vi "Read DC meter.vi"(6 "No of readings":i32=1, 7 "abort reference":refnum<vi>, 8 "error in (no error)":errorcluster, 11 "DC meter":T1={"DC meter type"=enum."H/A/K 3458", "DC meter VISA"="", "NPLC"=10.0, "status ref"=refnum}) -> (0 "error out":errorcluster, 2 "DC readings":dbl[](array[numeric]), 3 "DC meter out":T1={"DC meter type"=enum."H/A/K 3458", "DC meter VISA"="", "NPLC"=10.0, "status ref"=refnum})   [LabVIEW 2020]
doc: "Read selected number of values from the DC meter."
uses:
  Type definitions/DC meter.ctl
  Type definitions/DC meter type.ctl
  <vilib>/Utility/error.llb/Error Cluster From Error Code.vi
  external libraries/3458A Basic Driver/Public/Data/Read Measurement(Single Point).vi
  <vilib>/ErrorRing/Error Ring.xnode
  external libraries/Fluke 8508/Fluke 8508.lvlib
  external libraries/3458A Basic Driver/3458A Basic Driver.lvlib
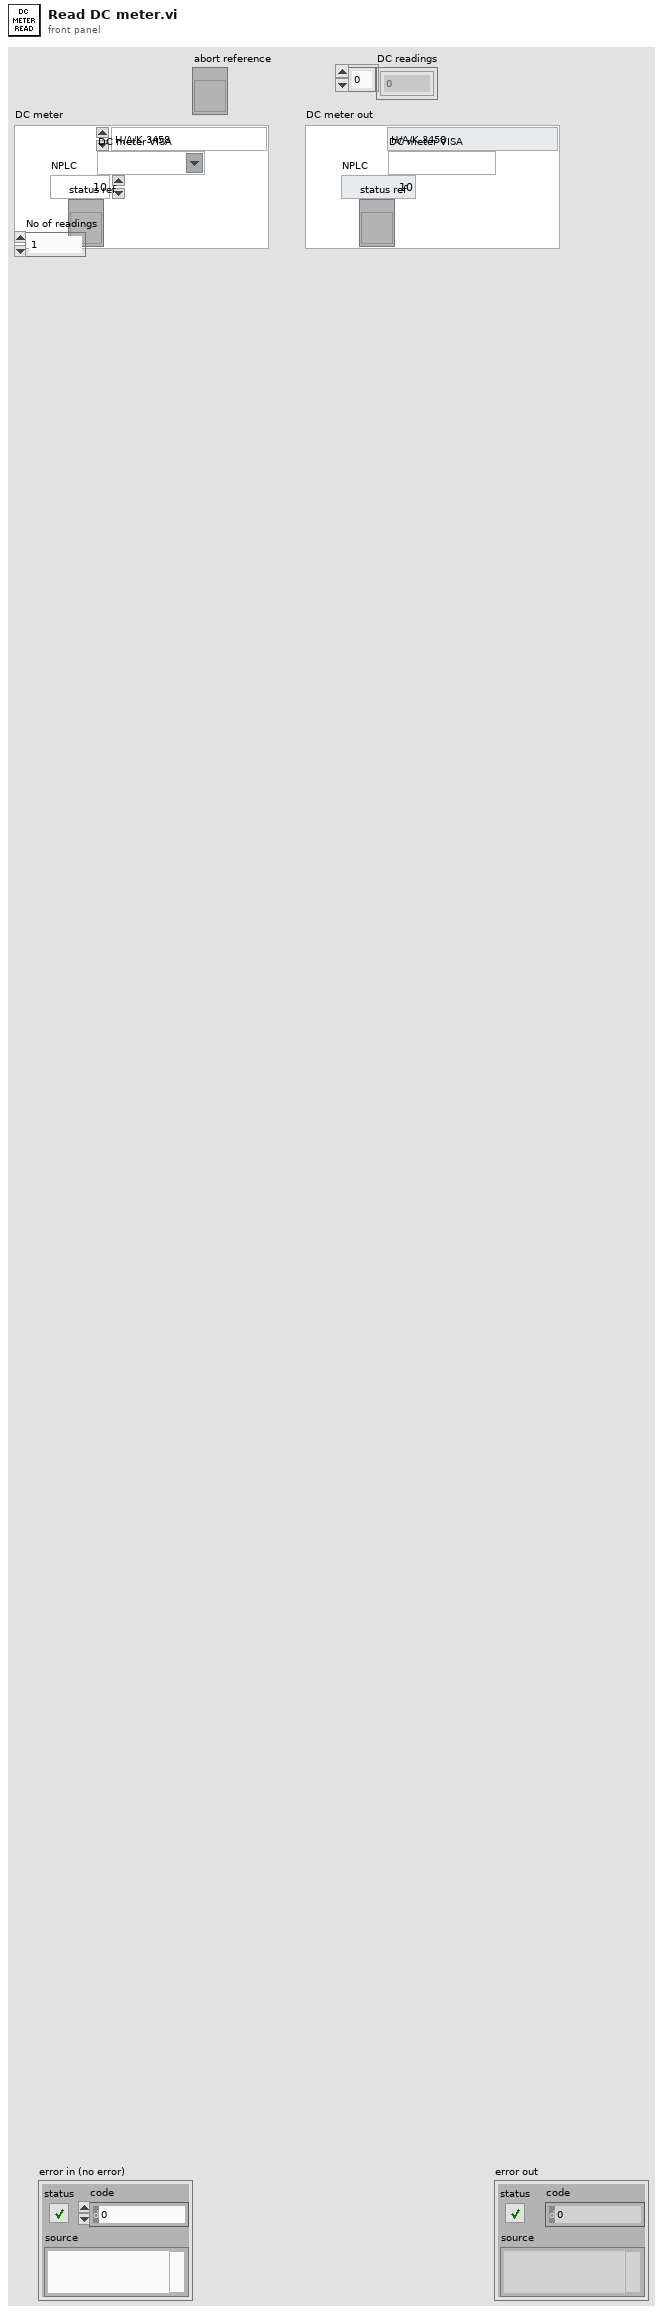
[diagram p1: front panel]
types:
  T1 = typedef "DC meter.ctl" = cluster{"DC meter type":T2, "DC meter VISA":refnum<visa-resource-name>, "NPLC":dbl, "status ref":refnum<vi>}
  T2 = typedef "DC meter type.ctl" = enum16{"H/A/K 3458", "Fluke 8508A", "dummy", "Keithley 2182"}
  T3 = cluster{"error":bool, "code":i32, "source":string}
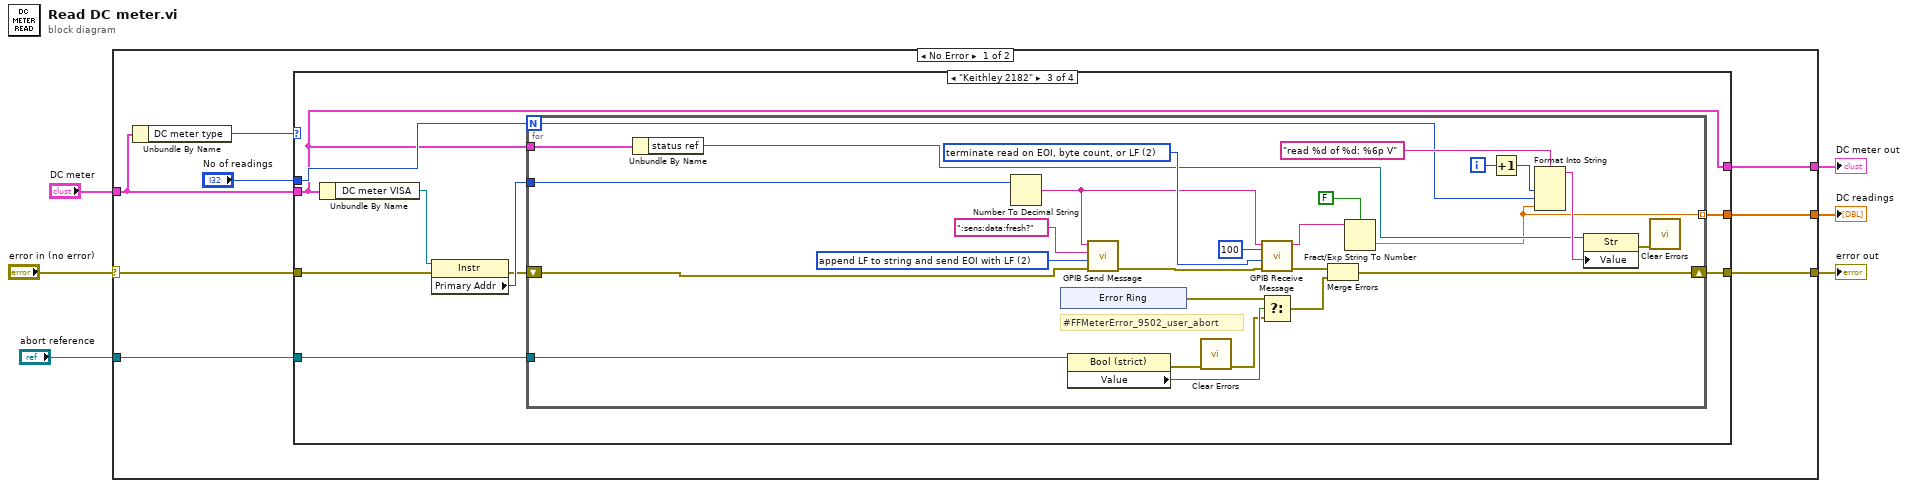
[diagram p0: block diagram]
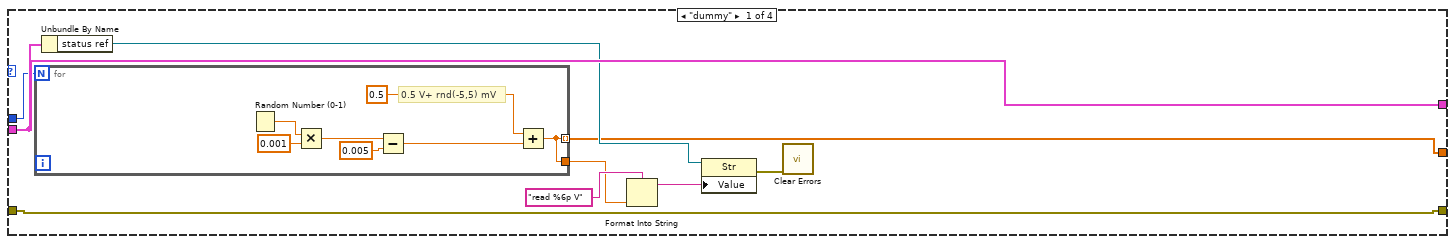
[diagram p2: hidden frame]
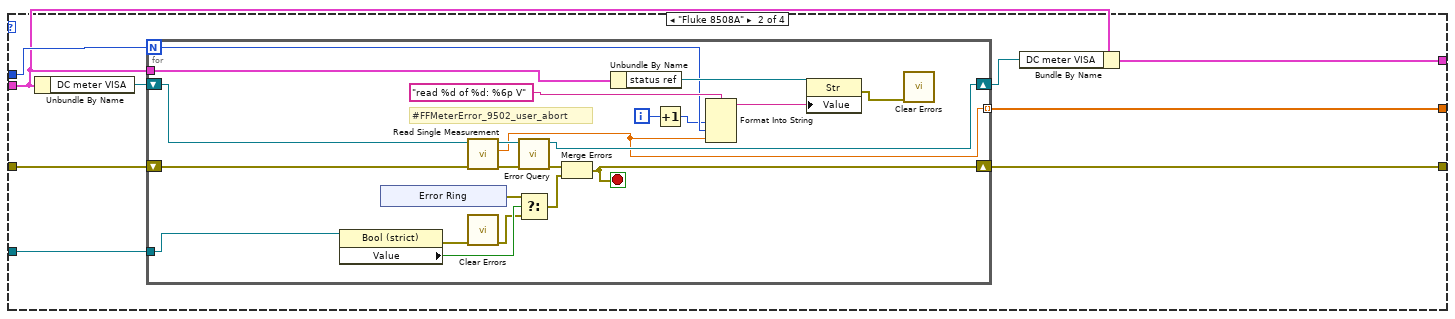
[diagram p3: hidden frame]
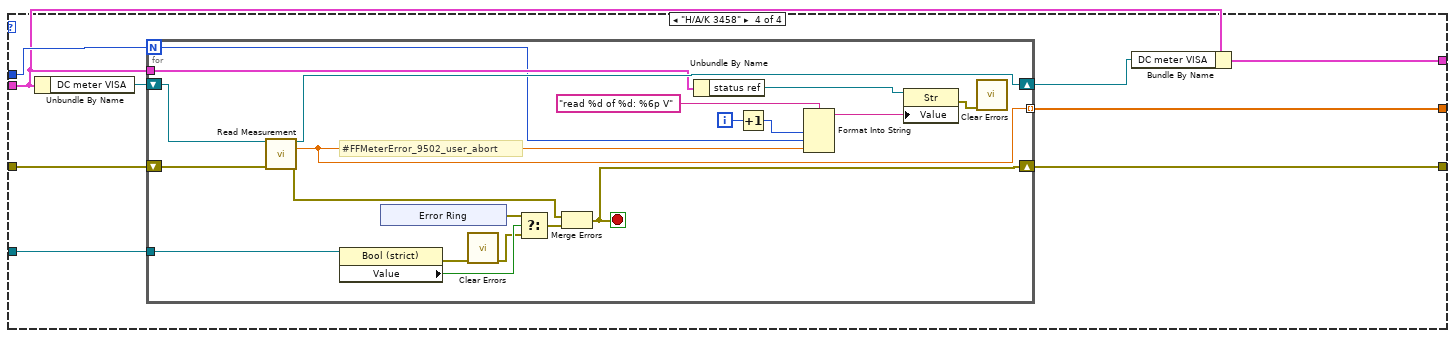
[diagram p4: hidden frame]
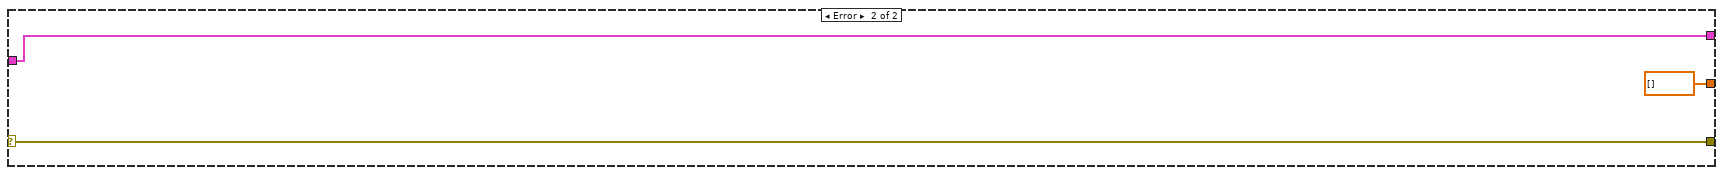
[diagram p5: hidden frame]
diagram:
  n1 = case shown="No Error" "error in (no error)" {
    selector: "error in (no error)" -> [w10 w144]
    tunnel: [w14 w144] -> w6
    tunnel: "DC meter" -> [w12 w143]
    tunnel: [w9 w143] -> w4
    tunnel: [w11 dbl[] [] ("Measurements")] -> w3
    tunnel: "abort reference" -> [w8 _]
    frame No Error {
      n2 = Unbundle By Name(w12) -> ("DC meter type"=w13:T2)
      n3 = case shown="\"Keithley 2182\"" w13 {
        tunnel: w10 -> [w23 w39 w74 w116]
        tunnel: [w23 w36 w71 w115] -> w14
        tunnel: w12 -> [w19 w33 w68 w110]
        tunnel: [w19 w37 w68 w109] -> w9
        tunnel: [w16 w32 w67 w113] -> w11
        tunnel: "No of readings" -> [w17 w34 w70 w112]
        tunnel: w8 -> [_ w31 w69 w108]
        frame "dummy" {
          n4 = for {
            N: w17 -> [_]
            tunnel: [w24] -> w16 mode=indexing
            tunnel: [w24] -> w15
            # "0.5 V+ rnd(-5,5) mV"
            n5 = Random Number (0-1)() -> (number: 0 to 1=w30:dbl)
            n6 = Multiply(x=w30, y=0.001) -> (x*y=w28:dbl)
            n7 = Subtract(x=w28, y=0.005) -> (x-y=w26:dbl)
            n8 = Add(x=0.5, y=w26) -> (x+y=w24:dbl)
          }
          n9 = Unbundle By Name(w19) -> ("status ref"=w18:refnum<vi>)
          n10 = Format Into String(format string="read %6p V", w15) -> (resulting string=w22:string)  [unwired: 2 in, 1 out]
          n11 = property class="Str"(reference=w18, "Value"=w22) -> (error out=w20:errorcluster)  [unwired: 1 in, 1 out]
          n12 = call <vilib>:"Clear Errors.vi"("error in (no error)"=w20) -> ()  [unwired: 5 in, 2 out]
        }
        frame "Fluke 8508A" {
          n13 = Unbundle By Name(w33) -> ("DC meter VISA"=w38:refnum<visa-resource-name>)
          n14 = for {
            N: w34 -> [w43]
            tunnel: [w44] -> w32 mode=indexing
            shift-right: [w40] -> w36
            shift-left: w39 -> [w61]
            shift-right: [w57] -> w35
            shift-left: w38 -> [w60]
            tunnel: w33 -> [w53]
            tunnel: w31 -> [w46]
            i -> [w42]
            stop <- w40 stop-if-true
            # "#FFMeterError_9502_user_abort"
            n15 = property class="Bool (strict)"(reference=w46) -> (error out=w51:errorcluster, "Value"=w50:bool)  [unwired: 1 in, 1 out]
            n16 = xnode "Error Ring"() -> ("error out"=w49:errorcluster)
            n17 = call "Read Single Measurement.vi"("error in (no error)"=w61, "VISA resource name"=w60) -> ("error out"=w59:errorcluster, "Measurement"=w44:dbl, "VISA resource name out"=w58:refnum<visa-resource-name>)  [unwired: 7 in]
            n18 = call <vilib>:"Clear Errors.vi"("error in (no error)"=w51) -> ("error out"=w48:errorcluster)  [unwired: 5 in, 1 out]
            n19 = call "Error Query.vi"("error in (no error)"=w59, "VISA resource name"=w58) -> ("error out"=w45:errorcluster, "VISA resource name out"=w57:refnum<visa-resource-name>)  [unwired: 6 in, 2 out]
            n20 = Select(t=w49, s=w50, f=w48) -> (s? t:f=w47:errorcluster)
            n21 = Merge Errors(w45, w47) -> (w40:errorcluster)
            n22 = Unbundle By Name(w53) -> ("status ref"=w56:refnum<vi>)
            n23 = Increment(x=w42) -> (x+1=w41:i32)
            n24 = Format Into String(format string="read %d of %d: %6p V", w41, w43, w44) -> (resulting string=w52:string)  [unwired: 2 in, 1 out]
            n25 = property class="Str"(reference=w56, "Value"=w52) -> (error out=w55:errorcluster)  [unwired: 1 in, 1 out]
            n26 = call <vilib>:"Clear Errors.vi"("error in (no error)"=w55) -> ()  [unwired: 5 in, 2 out]
          }
          n27 = Bundle By Name(cluster=w33, "DC meter VISA"=w35) -> (w37:T1)
        }
        frame "Keithley 2182" {
          n28 = Unbundle By Name(w68) -> ("DC meter VISA"=w75:refnum<visa-resource-name>)
          n29 = property class="Instr"(reference=w75, error in=w74) -> (error out=w72:errorcluster, "Primary Addr"=w73:u16)  [unwired: 1 out]
          n30 = for {
            N: w70 -> [w78]
            tunnel: w73 -> [w102]
            shift-right: [w86] -> w71
            shift-left: w72 -> [w101]
            tunnel: w69 -> [w85]
            tunnel: w68 -> [w77]
            tunnel: [w76] -> w67 mode=indexing
            i -> [w79]
            w96 = 2 items=["terminate read on EOI or byte count", "terminate read on EOI, byte count, or CR", "terminate read on EOI, byte count, or LF"] ("read mode")
            w98 = 2 items=["send EOI with last character of string", "append CR to string and send EOI with CR", "append LF to string and send EOI with LF", "append CR LF to string and send EOI with LF", "append CR to string but do not send EOI", "append LF to string but do not send EOI", "append CR LF to string but do not send EOI", "do not send EOI"] ("write mode (set END:0)")
            # "#FFMeterError_9502_user_abort"
            n31 = Unbundle By Name(w77) -> ("status ref"=w83:refnum<vi>)
            n32 = Number To Decimal String(number=w102) -> (decimal integer string=w94:string)  [unwired: 1 in]
            n33 = xnode "Error Ring"() -> ("error out"=w89:errorcluster)
            n34 = property class="Bool (strict)"(reference=w85) -> (error out=w91:errorcluster, "Value"=w90:bool)  [unwired: 1 in, 1 out]
            n35 = call "GPIB Send Message.vi"("address string"=w94, "write buffer"=":sens:data:fresh?", "write mode (set END:0)"=w98, "error in"=w101) -> ("error out"=w100:T3)  [unwired: 3 in, 2 out]
            n36 = call <vilib>:"Clear Errors.vi"("error in (no error)"=w91) -> ("error out"=w88:errorcluster)  [unwired: 5 in, 1 out]
            n37 = call "GPIB Receive Message.vi"("address string"=w94, "byte count"=100, "read mode"=w96, "error in"=w100) -> ("read buffer"=w93:string, "error out"=w87:T3)  [unwired: 3 in, 1 out]
            n38 = Select(t=w89, s=w90, f=w88) -> (s? t:f=w92:errorcluster)
            n39 = Merge Errors(w87, w92) -> (w86:errorcluster)
            n40 = Fract/Exp String To Number(use system decimal point (T)=FALSE, string=w93) -> (number=w76:dbl)  [unwired: 2 in, 1 out]
            n41 = Increment(x=w79) -> (x+1=w81:i32)
            n42 = Format Into String(format string="read %d of %d: %6p V", w81, w78, w76) -> (resulting string=w84:string)  [unwired: 2 in, 1 out]
            n43 = property class="Str"(reference=w83, "Value"=w84) -> (error out=w82:errorcluster)  [unwired: 1 in, 1 out]
            n44 = call <vilib>:"Clear Errors.vi"("error in (no error)"=w82) -> ()  [unwired: 5 in, 2 out]
          }
        }
        frame "H/A/K 3458" {
          n45 = Unbundle By Name(w110) -> ("DC meter VISA"=w114:refnum<visa-resource-name>)
          n46 = for {
            N: w112 -> [w119]
            tunnel: [w120] -> w113 mode=indexing
            shift-right: [w121] -> w115
            shift-left: w116 -> [w136]
            shift-right: [w130] -> w111
            shift-left: w114 -> [w135]
            tunnel: w110 -> [w129]
            tunnel: w108 -> [w124]
            i -> [w118]
            stop <- w121 stop-if-true
            # "#FFMeterError_9502_user_abort"
            n47 = call-poly "Read Measurement.vi"("VISA resource name"=w135, "error in (no error)"=w136) -> ("VISA resource name out"=w130:refnum<visa-resource-name>, "Measurement"=w120:dbl, "error out"=w123:errorcluster)  [unwired: 11 in]
            n48 = property class="Bool (strict)"(reference=w124) -> (error out=w128:errorcluster, "Value"=w127:bool)  [unwired: 1 in, 1 out]
            n49 = xnode "Error Ring"() -> ("error out"=w126:errorcluster)
            n50 = call <vilib>:"Clear Errors.vi"("error in (no error)"=w128) -> ("error out"=w125:errorcluster)  [unwired: 5 in, 1 out]
            n51 = Select(t=w126, s=w127, f=w125) -> (s? t:f=w122:errorcluster)
            n52 = Merge Errors(w123, w122) -> (w121:errorcluster)
            n53 = Unbundle By Name(w129) -> ("status ref"=w133:refnum<vi>)
            n54 = Increment(x=w118) -> (x+1=w117:i32)
            n55 = Format Into String(format string="read %d of %d: %6p V", w117, w119, w120) -> (resulting string=w134:string)  [unwired: 2 in, 1 out]
            n56 = property class="Str"(reference=w133, "Value"=w134) -> (error out=w132:errorcluster)  [unwired: 1 in, 1 out]
            n57 = call <vilib>:"Clear Errors.vi"("error in (no error)"=w132) -> ()  [unwired: 5 in, 2 out]
          }
          n58 = Bundle By Name(cluster=w110, "DC meter VISA"=w111) -> (w109:T1)
        }
      }
    }
    frame Error {
    }
  }
  "error out" <- w6
  "DC meter out" <- w4
  "DC readings" <- w3
